vi "DWSPT5_Open232.vi"(8 "error in (no error)":errorcluster, 10 "baud rate (9600)":u32=9600, 11 "VISA resource name":refnum<visa-resource-name>) -> (0 "error out":errorcluster, 3 "status":bool)   [LabVIEW 2017]
uses:
  <vilib>/Instr/_visa.llb/VISA Configure Serial Port (Instr).vi
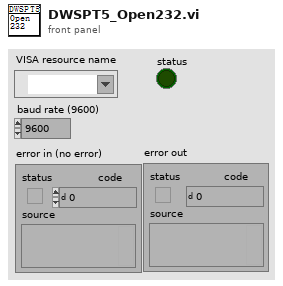
[diagram p1: front panel]
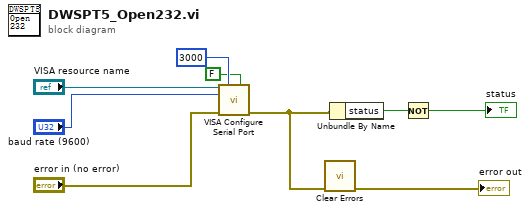
[diagram p0: block diagram]
diagram:
  n1 = call-poly "VISA Configure Serial Port"("VISA resource name"="VISA resource name", "timeout (10sec)"=u32 3000, "Enable Termination\nChar (T)"=FALSE ("Enable Termination\nChar (T)"), "baud rate (9600)"="baud rate (9600)", "error in (no error)"="error in (no error)") -> ("error out"=w6:errorcluster)  [unwired: 9 in, 1 out]
  n2 = call <vilib>:"Clear Errors.vi"("error in (no error)"=w6) -> ("error out"=→"error out":errorcluster)  [unwired: 5 in, 1 out]
  n3 = Unbundle By Name(w6) -> ("status"=w4:bool)
  n4 = Not(x=w4) -> (.not. x?=→"status":bool)
